vi "ECSensor.vi"() -> ()   [LabVIEW 2024]
uses:
  Driver/CTIPicoVISA.lvlib
panel:
  out "Identity":T1
  out "Value":u16(graph)
  in  "GroveConnector":enum16{"A0", "A1", "A2"}(ring)
  in  "stop":bool
  in  "VISA resource name in":refnum<visa-resource-name>="COM7"
  out "error out":errorcluster
  # "https://wiki.seeedstudio.com/Grove-EC-Sensor-kit/"
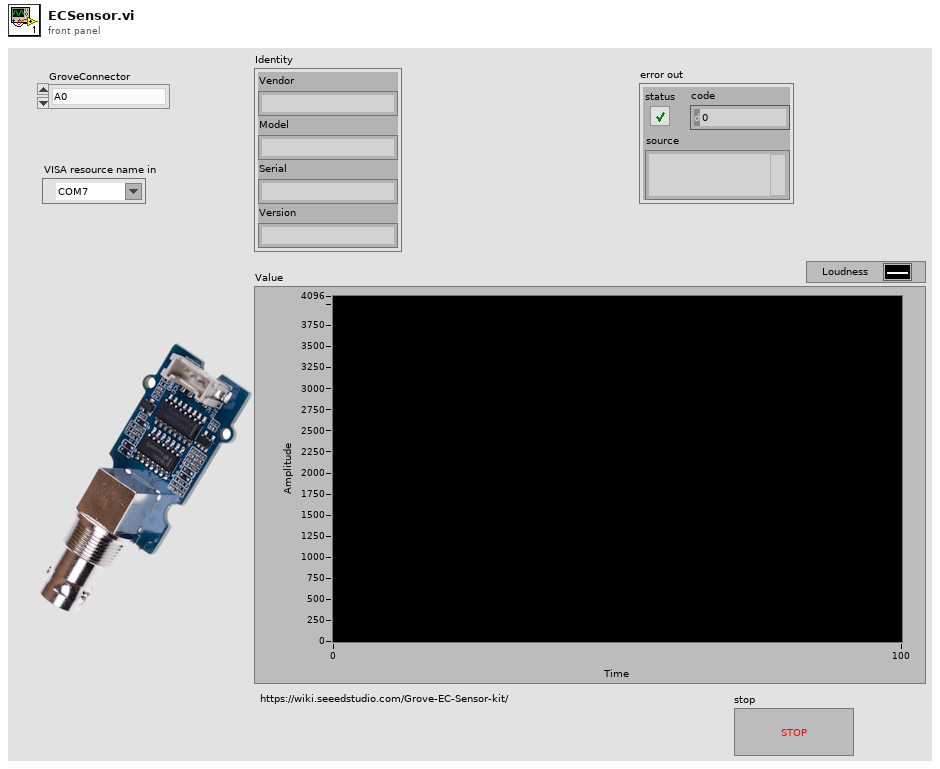
[diagram p1: front panel]
types:
  T1 = cluster{"Vendor":string, "Model":string, "Serial":string, "Version":string}
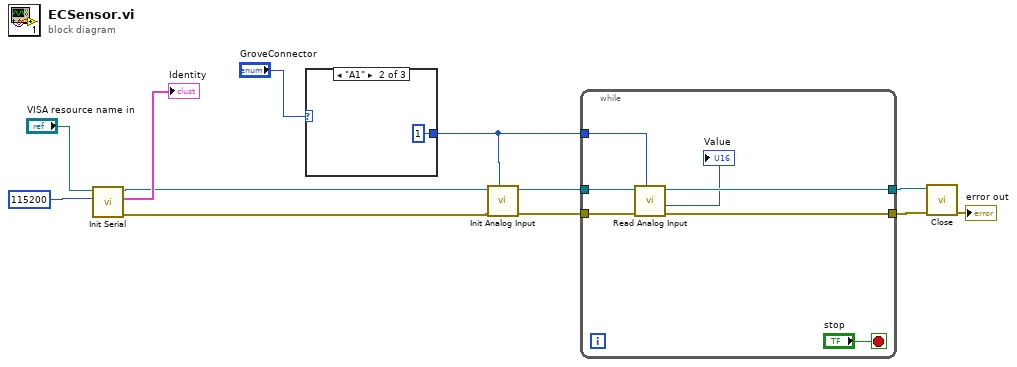
[diagram p0: block diagram]
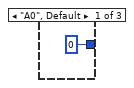
[diagram p2: hidden frame]
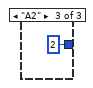
[diagram p3: hidden frame]
diagram:
  n1 = call "Init Serial.vi"("Baud (115200)"=u32 115200, "VISA resource name in"="VISA resource name in") -> ("error out"=w5:errorcluster, "Identity"=→"Identity":T1, "VISA resource name Out"=w6:refnum<visa-resource-name>)  [unwired: 7 in]
  n2 = case shown="\"A1\"" "GroveConnector" {
    tunnel: [0 ("GPIO") 1 ("GPIO") 2 ("GPIO")] -> w8
    frame "A0", Default {
    }
    frame "A1" {
    }
    frame "A2" {
    }
  }
  n3 = call "Init Analog Input.vi"("ADC"=w8, "error in (no error)"=w5, "VISA resource name in"=w6) -> ("error out"=w4:errorcluster, "VISA resource name"=w9:refnum<visa-resource-name>)  [unwired: 7 in]
  n4 = while {
    tunnel: w9 -> [w20]
    tunnel: w8 -> [w19]
    tunnel: [w18] -> w3
    tunnel: [w16] -> w2
    tunnel: w4 -> [w21]
    stop <- "stop" stop-if-true
    n5 = call "Read Analog Input.vi"("ADC"=w19, "error in (no error)"=w21, "VISA resource name in"=w20) -> ("error out"=w16:errorcluster, "Value"=→"Value":u16, "VISA resource name"=w18:refnum<visa-resource-name>)  [unwired: 6 in]
  }
  n6 = call "Close.vi"("error in (no error)"=w2, "VISA resource name in"=w3) -> ("error out"=→"error out":errorcluster)  [unwired: 9 in]
